vi "subDFD_Get Error Message.vi"(8 "error in (no error)":errorcluster) -> (2 "Error Message":string)   [LabVIEW 2017]
uses:
  <vilib>/Utility/error.llb/DialogType.ctl
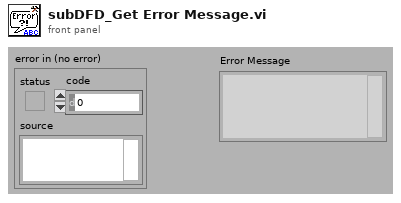
[diagram p1: front panel]
types:
  T1 = typedef "DialogType.ctl" = u16
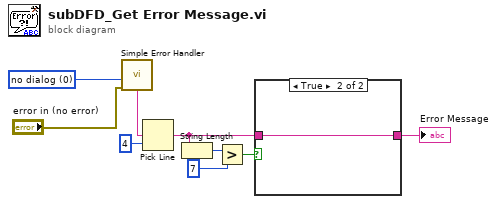
[diagram p0: block diagram]
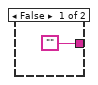
[diagram p2: hidden frame]
diagram:
  w9 = T1 0 items=["no dialog", "OK message", "continue or stop message", "OK message + warnings", "continue/stop + warnings"] ("type of dialog (OK msg:1)")
  n1 = call <vilib>:"Simple Error Handler.vi"("type of dialog (OK msg:1)"=w9, "error in (no error)"="error in (no error)") -> ("message"=w2:string)  [unwired: 7 out]
  n2 = Pick Line(multi-line string=w2, line index=4) -> (output string=w1:string)  [unwired: 1 out]
  n3 = String Length(string=w1) -> (length=w8:i32)
  n4 = Greater?(x=w8, y=7) -> (0:w6:bool)
  n5 = case shown="True" w6 {
    tunnel: ["" w11] -> w4
    tunnel: w1 -> [_ w11]
    frame False {
    }
    frame True {
    }
  }
  "Error Message" <- w4
